vi "Ref_2.vi"(0 "Control  Ch 3":refnum<vi>, 1 "Control  Ch 4":refnum<vi>, 2 "Control  Ch 5":refnum<vi>, 3 "Init_F":bool=TRUE, 4 "Control  Ch 6":refnum<vi>, 5 "Control  Ch 7":refnum<vi>, 6 "Control  Ch 8":refnum<vi>, 7 "error in":errorcluster, 8 "Control  Ch 2":refnum<vi>, 9 "Control  Ch 10":refnum<vi>, 10 "Control  Ch 1":refnum<vi>, 12 "Control  Ch 9":refnum<vi>) -> (16 "Control  Ch 10 out":refnum<vi>, 17 "Control  Ch 1 out":refnum<vi>, 18 "Control  Ch 9 out":refnum<vi>, 19 "Control  Ch 2 out":refnum<vi>, 21 "Control  Ch 8 out":refnum<vi>, 22 "Control  Ch 7 out":refnum<vi>, 23 "Control  Ch 6 out":refnum<vi>, 24 "Control  Ch 5 out":refnum<vi>, 25 "Control  Ch 4 out":refnum<vi>, 26 "Control  Ch 3 out":refnum<vi>, 27 "error out":errorcluster)   [LabVIEW 2010]
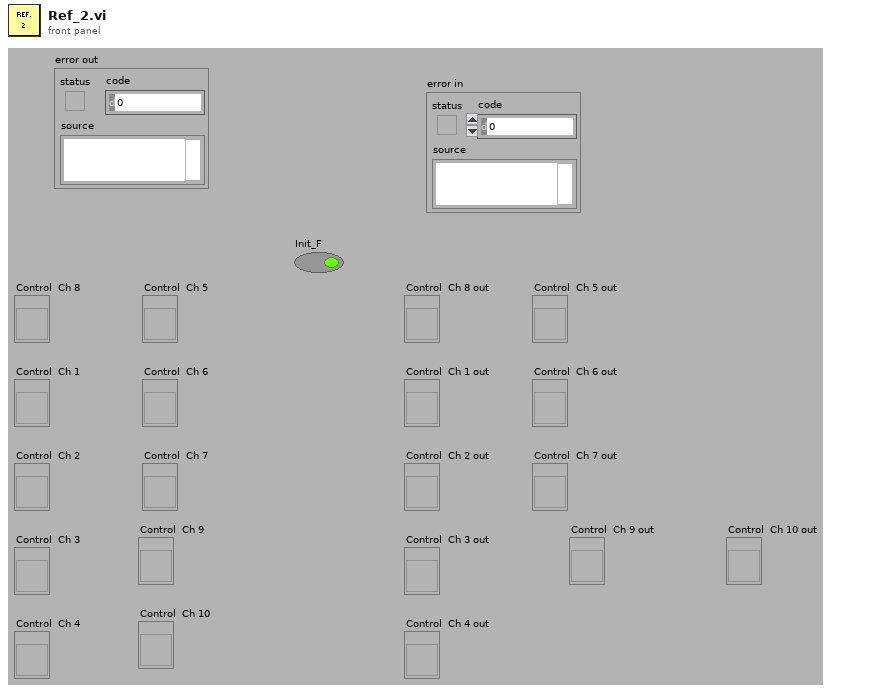
[diagram p1: front panel]
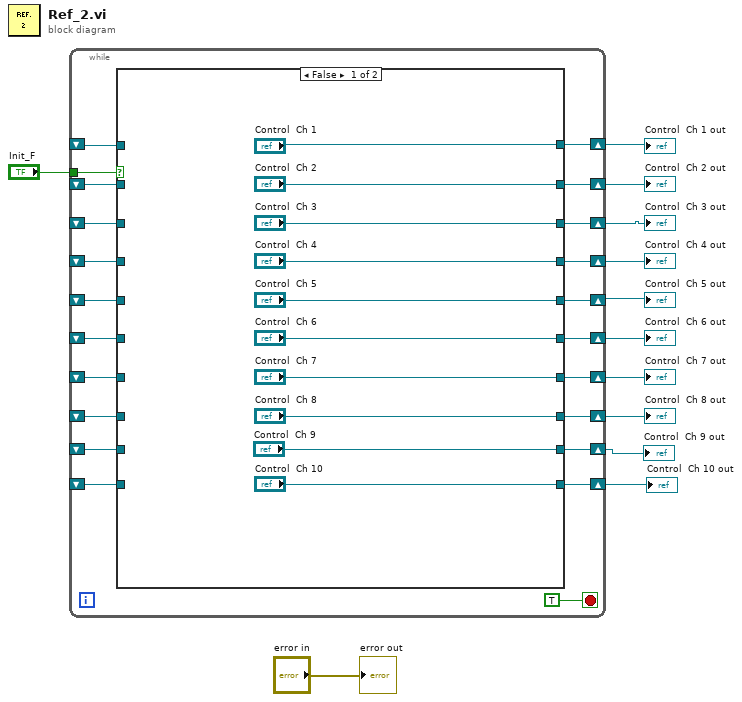
[diagram p0: block diagram]
diagram:
  n1 = while {
    shift-right: [w33] -> w10
    shift-left: _ -> [w32]
    tunnel: "Init_F" -> [w31]
    shift-right: [w30] -> w9
    shift-left: _ -> [w23]
    shift-right: [w29] -> w6
    shift-left: _ -> [w22]
    shift-right: [w28] -> w8
    shift-left: _ -> [w17]
    shift-right: [w27] -> w7
    shift-left: _ -> [w21]
    shift-right: [w26] -> w5
    shift-left: _ -> [w20]
    shift-right: [w25] -> w4
    shift-left: _ -> [w19]
    shift-right: [w24] -> w3
    shift-left: _ -> [w18]
    shift-right: [w16] -> w2
    shift-left: _ -> [w14]
    shift-right: [w15] -> w1
    shift-left: _ -> [w13]
    stop <- TRUE stop-if-true
    n2 = case shown="False" w31 {
      tunnel: ["Control  Ch 1" w54] -> w33
      tunnel: w32 -> [_ w54]
      tunnel: ["Control  Ch 2" w47] -> w30
      tunnel: ["Control  Ch 3" w48] -> w29
      tunnel: ["Control  Ch 4" w49] -> w28
      tunnel: ["Control  Ch 5" w50] -> w27
      tunnel: ["Control  Ch 6" w51] -> w26
      tunnel: ["Control  Ch 7" w52] -> w25
      tunnel: ["Control  Ch 8" w53] -> w24
      tunnel: w23 -> [_ w47]
      tunnel: w22 -> [_ w48]
      tunnel: w21 -> [_ w50]
      tunnel: w20 -> [_ w51]
      tunnel: w19 -> [_ w52]
      tunnel: w18 -> [_ w53]
      tunnel: w17 -> [_ w49]
      tunnel: ["Control  Ch 9" w46] -> w16
      tunnel: ["Control  Ch 10" w45] -> w15
      tunnel: w14 -> [_ w46]
      tunnel: w13 -> [_ w45]
      frame False {
      }
      frame True {
      }
    }
  }
  "Control  Ch 8 out" <- w3
  "Control  Ch 7 out" <- w4
  "Control  Ch 6 out" <- w5
  "Control  Ch 5 out" <- w7
  "Control  Ch 4 out" <- w8
  "Control  Ch 3 out" <- w6
  "Control  Ch 2 out" <- w9
  "Control  Ch 1 out" <- w10
  "Control  Ch 9 out" <- w2
  "Control  Ch 10 out" <- w1
  "error out" <- "error in"
